vi "LJUD UE9RAW Feedback.vi"(5 "Comm Settings":T1={"Open LabJack "=TRUE, "Use USB"=TRUE, "IP Address"="192.168.1.209", "PortA"=52360, "PortB"=0}, 6 "Digital IN":T4, 8 "error in (no error)":errorcluster, 9 "Analog Outputs":T2={"DAC0"=0, "DAC1"=0, "Update DACs"=TRUE, "Enable DACs"=TRUE}, 10 "AIN Options":T5={"AINMask"=1, "AIN14Select"=128, "AIN15Select"=136, "ResolutionIndex"=12, "Settling Index"=0, "Bip/Gain (per CH)"=[8, 8, 8, 8, 8, 8, 8, 8, 8, 8, 8, 8, 8, 8, 8, 8]}, 11 "Handle In":i32) -> (0 "error out":errorcluster, 2 "Analog Inputs":u16[](array[numeric]), 3 "Handle Out":i32, 4 "Digital Out":T3)   [LabVIEW 2021]
panel:
  out "milliseconds":u32
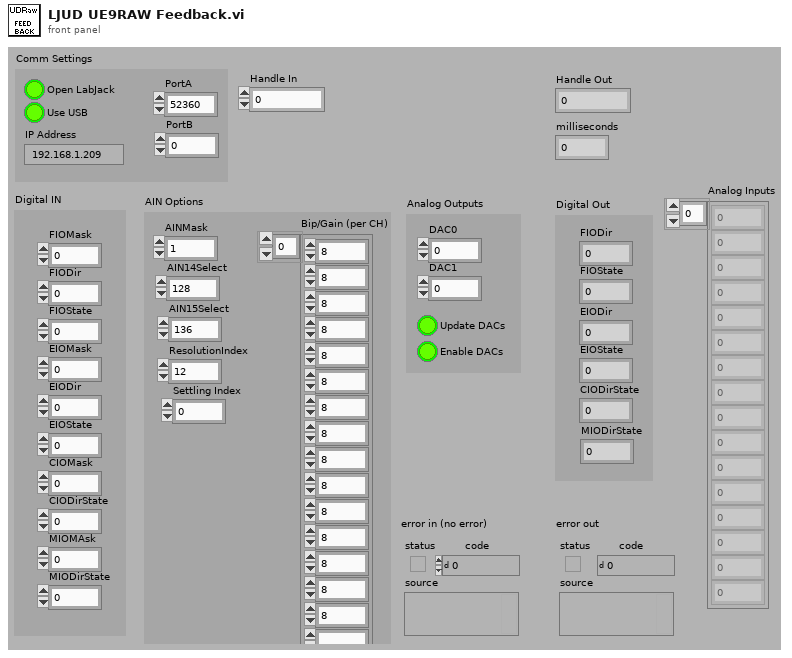
[diagram p1: front panel]
types:
  T1 = cluster{"Open LabJack ":bool, "Use USB":bool, "IP Address":string, "PortA":u16, "PortB":u16}
  T2 = cluster{"DAC0":u16, "DAC1":u16, "Update DACs":bool, "Enable DACs":bool}
  T3 = cluster{"FIODir":u8, "FIOState":u8, "EIODir":u8, "EIOState":u8, "CIODirState":u8, "MIODirState":u8}
  T4 = cluster{"FIOMask":u8, "FIODir":u8, "FIOState":u8, "EIOMask":u8, "EIODir":u8, "EIOState":u8, "CIOMask":u8, "CIODirState":u8, "MIOMAsk":u8, "MIODirState":u8}
  T5 = cluster{"AINMask":u16, "AIN14Select":u8, "AIN15Select":u8, "ResolutionIndex":u8, "Settling Index":u8, "Bip/Gain (per CH)":u8[]}
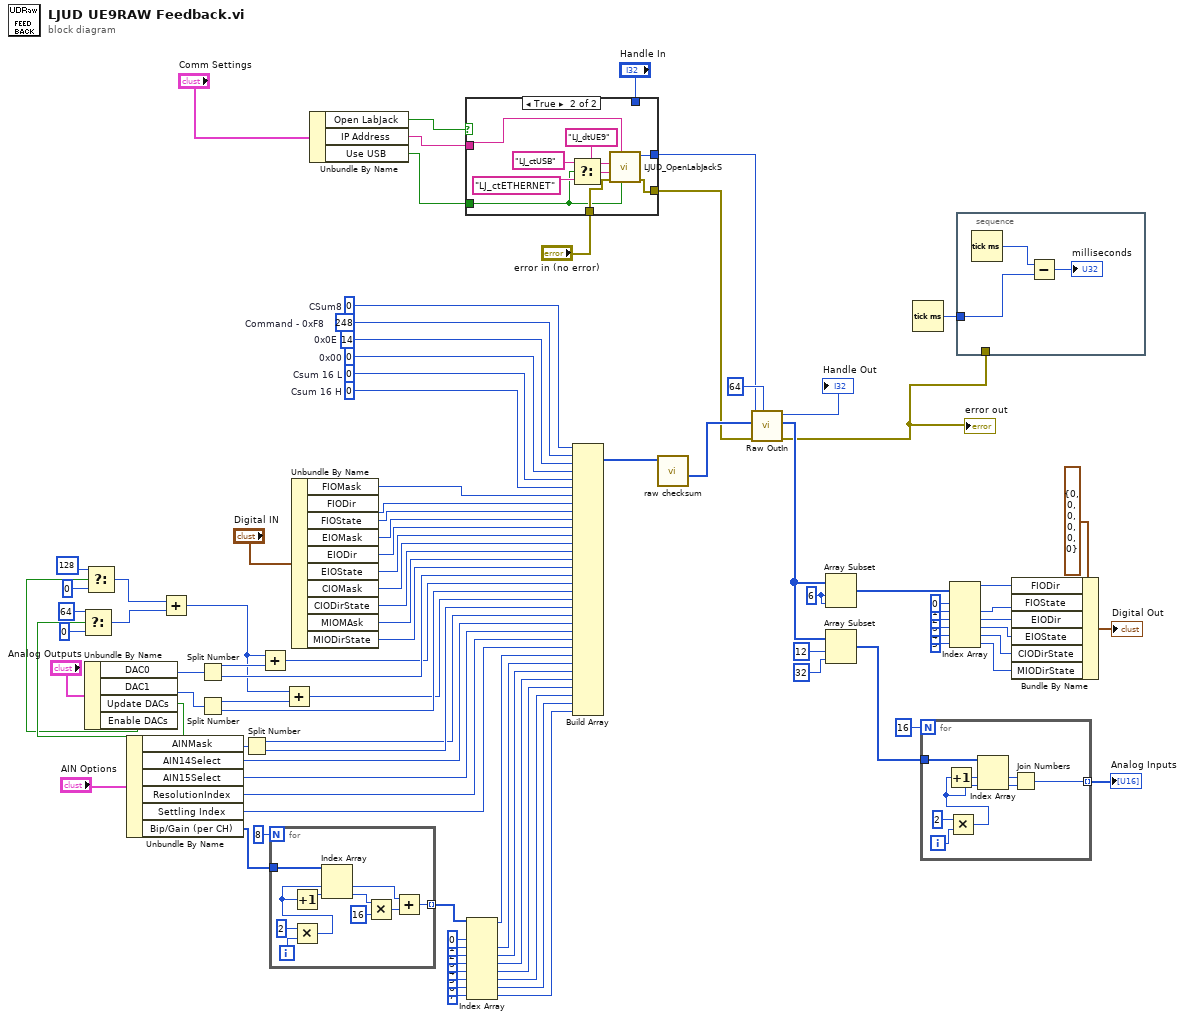
[diagram p0: block diagram]
diagram:
  w59 = 6 ("Array Index")
  w92 = u8 0  # Csum 16 H
  w93 = u8 0  # Csum 16 L
  w94 = u8 0  # 0x00
  w95 = u8 14  # 0x0E
  w96 = u8 0  # CSum8
  w98 = u8 248  # Command - 0xF8
  n1 = Unbundle By Name("Analog Outputs") -> ("DAC0"=w78:u16, "DAC1"=w77:u16, "Update DACs"=w18:bool, "Enable DACs"=w4:bool)
  n2 = Select(t=u8 64 ("x"), s=w18, f=u8 0 ("x")) -> (s? t:f=w2:u8)
  n3 = Select(t=u8 128 ("x"), s=w4, f=u8 0 ("x")) -> (s? t:f=w1:u8)
  n4 = Unbundle By Name("AIN Options") -> ("AINMask"=w74:u16, "AIN14Select"=w71:u8, "AIN15Select"=w70:u8, "ResolutionIndex"=w69:u8, "Settling Index"=w68:u8, "Bip/Gain (per CH)"=w39:u8[])
  n5 = Add(x=w1, y=w2) -> (x+y=w19:u8)
  n6 = Split Number(x=w78) -> (hi(x)=w27:u8, lo(x)=w76:u8)
  n7 = Split Number(x=w77) -> (hi(x)=w25:u8, lo(x)=w75:u8)
  n8 = Split Number(x=w74) -> (hi(x)=w72:u8, lo(x)=w73:u8)
  n9 = Add(x=w19, y=w27) -> (x+y=w26:u8)
  n10 = for {
    N: 8 -> [_]
    tunnel: w39 -> [w107]
    tunnel: [w99] -> w37 mode=indexing
    i -> [w106]
    n11 = Multiply(x=2, y=w106) -> (x*y=w103:i32)
    n12 = Increment(x=w103) -> (x+1=w102:i32)
    n13 = Index Array(array=w107, index #1=w103, index #2=w102) -> (element #1=w101:u8, element #2=w100:u8)
    n14 = Multiply(x=w100, y=16) -> (x*y=w104:i32)
    n15 = Add(x=w101, y=w104) -> (x+y=w99:i32)
  }
  n16 = Add(x=w19, y=w25) -> (x+y=w24:u8)
  n17 = Unbundle By Name("Digital IN") -> ("FIOMask"=w90:u8, "FIODir"=w89:u8, "FIOState"=w88:u8, "EIOMask"=w87:u8, "EIODir"=w86:u8, "EIOState"=w85:u8, "CIOMask"=w84:u8, "CIODirState"=w83:u8, "MIOMAsk"=w82:u8, "MIODirState"=w81:u8)
  n18 = Unbundle By Name("Comm Settings") -> ("Open LabJack"=w11:bool, "IP Address"=w12:string, "Use USB"=w10:bool)
  n19 = case shown="True" w11 {
    tunnel: w12 -> [_ w115]
    tunnel: "error in (no error)" -> [w110 w116]
    tunnel: [w110 w111] -> w8
    tunnel: [w109 w112] -> w9
    tunnel: w10 -> [_ w114]
    tunnel: "Handle In" -> [w109 _]
    frame False {
    }
    frame True {
      n20 = Select(t="LJ_ctUSB" ("ConnectionType"), s=w114, f="LJ_ctETHERNET" ("ConnectionType")) -> (s? t:f=w119:string)
      n21 = call "LJUD_OpenLabJackS.vi"("FirstFound"=w114, "Address"=w115, "error in"=w116, "ConnectionType"=w119, "DeviceType"="LJ_dtUE9") -> ("error out"=w111:errorcluster, "Handle"=w112:i32)  [unwired: 4 in, 1 out]
    }
  }
  n22 = Index Array(array=w37, index #1=0 ("Index"), index #2=1 ("Index"), index #3=2 ("Index"), index #4=3 ("Index"), index #5=4 ("Index"), index #6=5 ("Index"), index #7=6 ("Index"), index #8=7 ("Index")) -> (element #1=w36:i32, element #2=w35:i32, element #3=w34:i32, element #4=w33:i32, element #5=w32:i32, element #6=w31:i32, element #7=w30:i32, element #8=w29:i32)
  n23 = Build Array(w96, w98, w95, w94, w93, w92, w90, w89, w88, w87, w86, w85, w84, w83, w82, w81, w76, w26, w75, w24, w73, w72, w71, w70, w69, w68, w36, w35, w34, w33, w32, w31, w30, w29) -> (w97:i32[])
  n24 = call "raw checksum.vi"("Array"=w97) -> ("Array Output"=w17:u8[])  [unwired: 3 in, 7 out]
  n25 = call "Raw OutIn.vi"("# of bytes to read in"=64 ("# of bytes to read"), "error in"=w8, "Raw Out"=w17, "Handle In"=w9) -> ("error out"=w13:errorcluster, "Raw In"=w16:u8[], "Handle Out"=→"Handle Out":i32)  [unwired: 4 in, 1 out]
  "error out" <- w13
  n26 = Array Subset(array=w16, index=w59, length=w59) -> (w56:u8[])
  n27 = Array Subset(array=w16, index=12 ("Array Index"), length=32 ("Array Length")) -> (w43:u8[])
  n28 = Tick Count (ms)() -> (millisecond timer value=w23:u32)
  n29 = for {
    N: 16 -> [_]
    tunnel: w43 -> [w125]
    tunnel: [w120] -> w22 mode=indexing
    i -> [w127]
    n30 = Multiply(x=2, y=w127) -> (x*y=w123:i32)
    n31 = Increment(x=w123) -> (x+1=w124:i32)
    n32 = Index Array(array=w125, index #1=w124, index #2=w123) -> (element #1=w122:u8, element #2=w121:u8)
    n33 = Join Numbers(hi=w122, lo=w121) -> ((hi.lo)=w120:u16)
  }
  "Analog Inputs" <- w22
  n34 = Index Array(array=w56, index #1=0 ("Index"), index #2=1 ("Index"), index #3=2 ("Index"), index #4=3 ("Index"), index #5=4 ("Index"), index #6=5 ("Index")) -> (element #1=w49:u8, element #2=w48:u8, element #3=w47:u8, element #4=w46:u8, element #5=w45:u8, element #6=w44:u8)
  n35 = stacked-sequence {
    tunnel: w23 -> [w130]
    tunnel: w13 -> [_]
    frame #0 {
      n36 = Tick Count (ms)() -> (millisecond timer value=w129:u32)
      n37 = Subtract(x=w129, y=w130) -> (x-y=→"milliseconds":u32)
    }
  }
  n38 = Bundle By Name(cluster=T3 {"FIODir"=0, "FIOState"=0, "EIODir"=0, "EIOState"=0, "CIODirState"=0, "MIODirState"=0} ("Digital Out"), "FIODir"=w49, "FIOState"=w48, "EIODir"=w47, "EIOState"=w46, "CIODirState"=w45, "MIODirState"=w44) -> (→"Digital Out":T3)
